vi "REPORT_DATES_date_time_selectors_get_init_values.vi"() -> (0 "time_end":timestamp, 1 "time_start":timestamp, 2 "date_end":timestamp, 3 "date_start":timestamp)   [LabVIEW 2019]
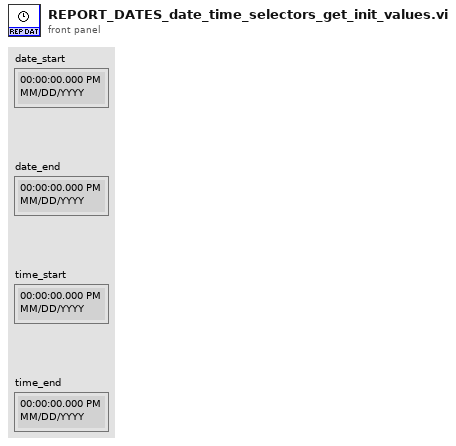
[diagram p1: front panel]
types:
  T1 = typedef "LVDateTimeRec.ctl" = cluster{"fractional second":dbl, "second":i32, "minute":i32, "hour":i32, "day of month":i32, "month":i32, "year":i32, "day of week":i32, "day of year":i32, "DST":i32}
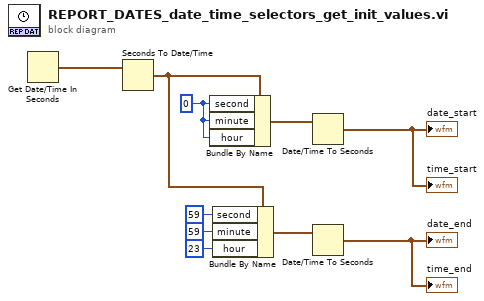
[diagram p0: block diagram]
diagram:
  w8 = 0 ("second")
  n1 = Get Date/Time In Seconds() -> (seconds since 1Jan1904=w9:timestamp)
  n2 = Seconds To Date/Time(time stamp (now)=w9) -> (date time rec=w1:T1)  [unwired: 1 in]
  n3 = Bundle By Name(cluster=w1, "second"=w8, "minute"=w8, "hour"=w8) -> (w10:T1)
  n4 = Bundle By Name(cluster=w1, "second"=59, "minute"=59, "hour"=23) -> (w7:T1)
  n5 = Date/Time To Seconds(2:w10) -> (0:→"date_start" →"time_start":timestamp)  [unwired: 1 in]
  n6 = Date/Time To Seconds(2:w7) -> (0:→"date_end" →"time_end":timestamp)  [unwired: 1 in]
